vi "6 - Sequência de Fibonacci.vi"() -> ()   [LabVIEW 2020]
panel:
  in  "N-ésimo número":dbl
  out "Memória de Número":dbl
  out "Número de Fibonacci":dbl format="%#_15f"
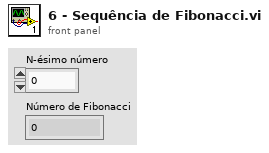
[diagram p1: front panel]
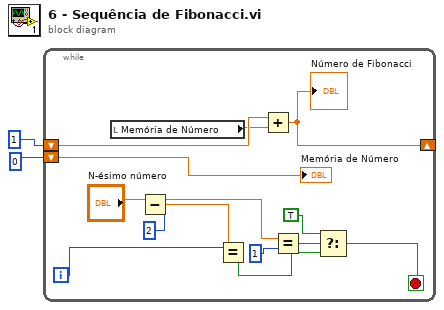
[diagram p0: block diagram]
diagram:
  n1 = while {
    shift-right: [w12] -> _
    shift-left: 1 -> [w14]
    shift-left: 0 -> [w15]
    i -> [w11]
    stop <- w3 stop-if-true
    n2 = local read "Memória de Número"() -> (w13:dbl)
    n3 = Subtract(x="N-ésimo número", y=2) -> (x-y=w9:dbl)
    n4 = Equal?(x=w11, y=w9) -> (x = y?=w4:bool)
    n5 = Add(x=w14, y=w13) -> (x+y=w12:dbl)
    "Número de Fibonacci" <- w12
    n6 = Equal?(x="N-ésimo número", y=1) -> (x = y?=w8:bool)
    n7 = Select(t=TRUE, s=w8, f=w4) -> (s? t:f=w3:bool)
    "Memória de Número" <- w15
  }
